vi "TSC Material Boolean Type--constant.vi"() -> (2 "boolean types":string[](array[string]))   [LabVIEW 2021, in "Material SubVIs.lvlib"]
doc: "CONSTANT VI to hold the options for the Boolean Types for the buttons. This is used when coloring the UI to figure out how to apply the correct layers of six-color button options.\n\n<b>Code Developed By:</b> +\nDaniel Coons +\nTechnology Service Corporation +\nwww.tsc.com/atcs"
uses:
  Material SubVIs.lvlib
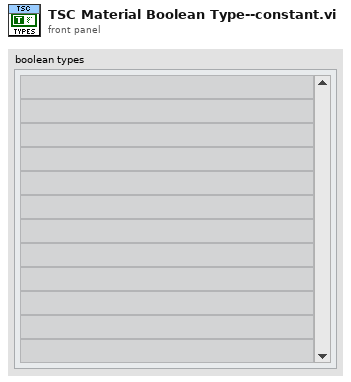
[diagram p1: front panel]
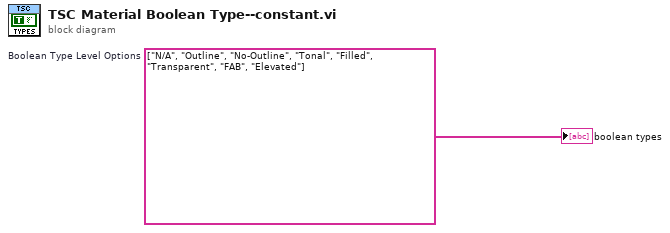
[diagram p0: block diagram]
diagram:
  w1 = string[] ["N/A", "Outline", "No-Outline", "Tonal", "Filled", "Transparent", "FAB", "Elevated"]  # Boolean Type Level Options
  "boolean types" <- w1
